vi "destroyPubDataUserEvents.vi"(8 "error in (no error)":errorcluster, 11 "PubSubDataEvent in":refnum<class "PubSubDataEvent.lvclass">) -> (0 "error out":errorcluster, 3 "PubSubDataEvent out":refnum<class "PubSubDataEvent.lvclass">)   [LabVIEW 2016, in "PubSubDataEvent.lvclass"]
uses:
  PubSubDataEvent.lvclass
  PubSubDataEvent.lvclass/PubSubDataEvent.ctl
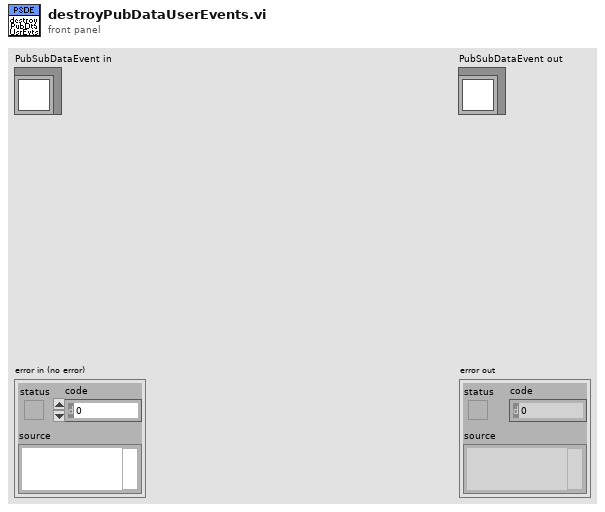
[diagram p1: front panel]
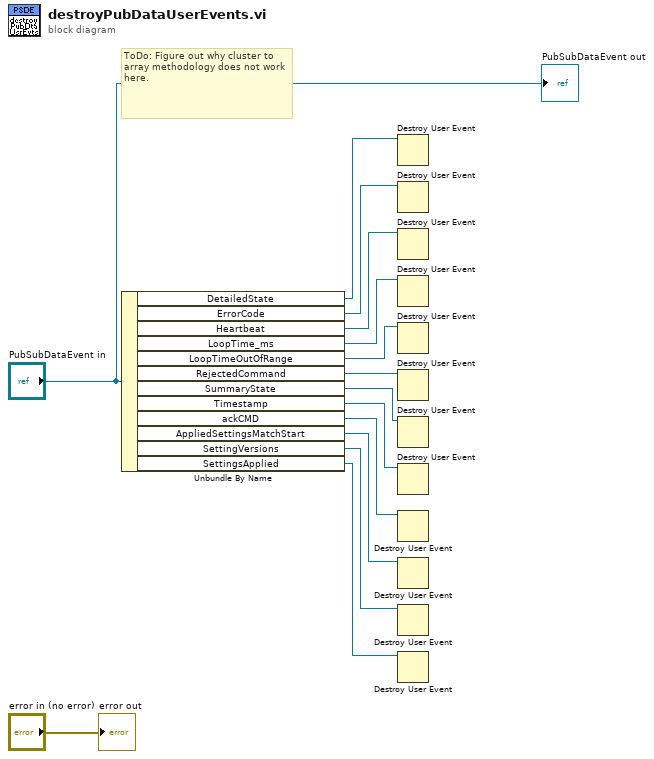
[diagram p0: block diagram]
diagram:
  # "ToDo: Figure out why cluster to array methodology does not work here."
  n1 = Unbundle By Name("PubSubDataEvent in") -> ("DetailedState"=w13:refnum<user-event>, "ErrorCode"=w12:refnum<user-event>, "Heartbeat"=w11:refnum<user-event>, "LoopTime_ms"=w10:refnum<user-event>, "LoopTimeOutOfRange"=w9:refnum<user-event>, "RejectedCommand"=w8:refnum<user-event>, "SummaryState"=w7:refnum<user-event>, "Timestamp"=w6:refnum<user-event>, "ackCMD"=w4:refnum<user-event>, "AppliedSettingsMatchStart"=w3:refnum<user-event>, "SettingVersions"=w2:refnum<user-event>, "SettingsApplied"=w1:refnum<user-event>)
  n2 = Destroy User Event(user event=w13) -> ()  [unwired: 1 in, 1 out]
  n3 = Destroy User Event(user event=w12) -> ()  [unwired: 1 in, 1 out]
  n4 = Destroy User Event(user event=w11) -> ()  [unwired: 1 in, 1 out]
  n5 = Destroy User Event(user event=w10) -> ()  [unwired: 1 in, 1 out]
  n6 = Destroy User Event(user event=w9) -> ()  [unwired: 1 in, 1 out]
  n7 = Destroy User Event(user event=w8) -> ()  [unwired: 1 in, 1 out]
  n8 = Destroy User Event(user event=w7) -> ()  [unwired: 1 in, 1 out]
  n9 = Destroy User Event(user event=w6) -> ()  [unwired: 1 in, 1 out]
  n10 = Destroy User Event(user event=w4) -> ()  [unwired: 1 in, 1 out]
  n11 = Destroy User Event(user event=w3) -> ()  [unwired: 1 in, 1 out]
  n12 = Destroy User Event(user event=w2) -> ()  [unwired: 1 in, 1 out]
  n13 = Destroy User Event(user event=w1) -> ()  [unwired: 1 in, 1 out]
  "error out" <- "error in (no error)"
  "PubSubDataEvent out" <- "PubSubDataEvent in"
